vi "DrawSeparator.vi"(7 "Collection in":refnum<class "Collection.lvclass">, 8 "error in (no error)":errorcluster, 9 "XPos":i16, 10 "Point":refnum<class "Point.lvclass">, 11 "Menu in":refnum<class "Menu.lvclass">) -> (0 "error out":errorcluster, 2 "rect":T1, 3 "Menu out":refnum<class "Menu.lvclass">, 5 "Collection out":refnum<class "Collection.lvclass">)   [LabVIEW 2021, in "Menu.lvlib" / "Menu.lvclass"]
uses:
  Menu.lvclass
  Picture2D/src/Point/Point.lvclass
  Picture2D/src/Collection/Collection.lvclass
  Picture2D/src/Line/Line.lvclass
  C:/GitHub/Picture2D/src/Shape/Shape.lvclass
  C:/GitHub/Picture2D/src/IDrawable/IDrawable.lvclass
  Picture2D/src/Text/Text.lvclass
  C:/GitHub/Picture2D/src/Picture2D/Picture2D.lvclass
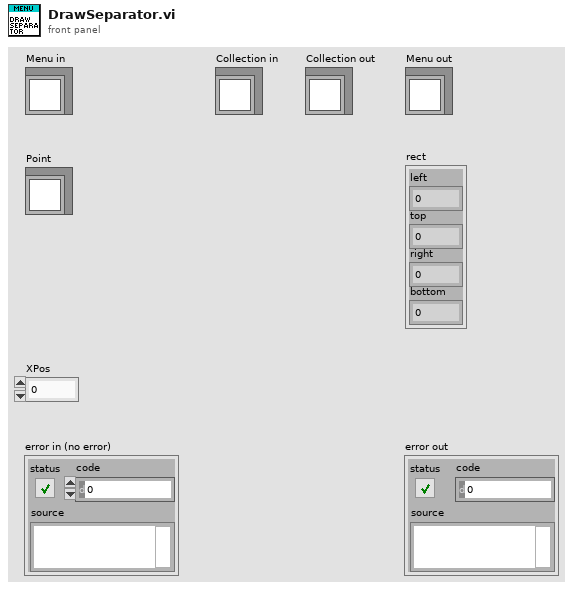
[diagram p1: front panel]
types:
  T1 = cluster{"left":i16, "top":i16, "right":i16, "bottom":i16}
  T2 = typedef "Menu.lvlib/Menu.lvclass/MenuColors.ctl" = cluster{"Text":refnum<class "Color.lvclass">, "HiliteText":refnum<class "Color.lvclass">, "Background":refnum<class "Color.lvclass">, "BorderColor":refnum<class "Color.lvclass">, "Hilite":refnum<class "Color.lvclass">}
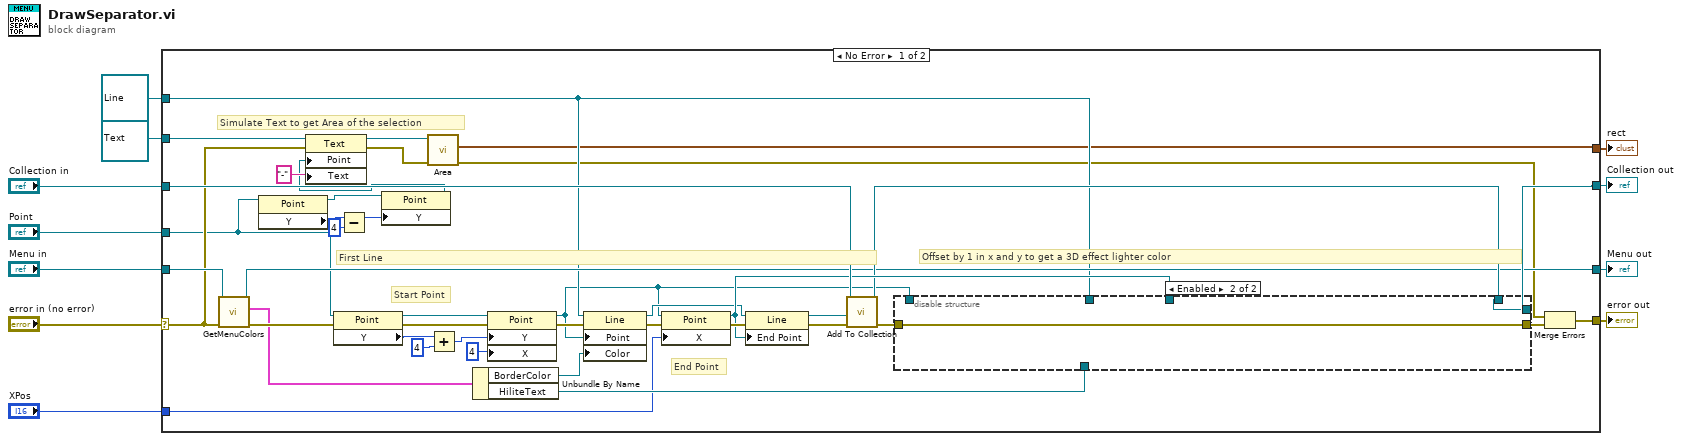
[diagram p0: block diagram]
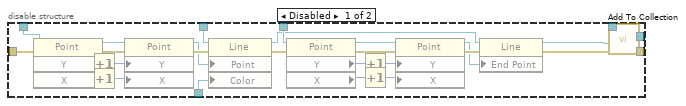
[diagram p2: hidden frame]
diagram:
  n1 = case shown="No Error" "error in (no error)" {
    selector: "error in (no error)" -> [w27 w83]
    tunnel: [w25 w83] -> w11
    tunnel: "XPos" -> [w45 _]
    tunnel: "Point" -> [w17 _]
    tunnel: [w19 _] -> w8
    tunnel: "Collection in" -> [w39 w84]
    tunnel: [w38 w84] -> w6
    tunnel: [w32 w85] -> w4
    tunnel: "Menu in" -> [w31 w85]
    tunnel: refnum<class "Line.lvclass"> refnum ("Picture2D.lvlib:Line") -> [w29 _]
    tunnel: refnum<class "Text.lvclass"> refnum ("Picture2D.lvlib:Text") -> [w28 _]
    frame No Error {
      # "End Point"
      # "Start Point"
      # "Simulate Text to get Area of the selection"
      # "First Line"
      # "Offset by 1 in x and y to get a 3D effect lighter color"
      n2 = call "GetMenuColors.vi"("error in (no error)"=w27, "Menu in"=w31) -> ("error out"=w33:errorcluster, "MenuColors"=w30:T2, "Menu out"=w32:refnum<class "Menu.lvclass">)  [unwired: 7 in]
      n3 = property class="Point"(reference=w17) -> (reference out=w15:refnum<class "Point.lvclass">, "Y"=w16:i16)  [unwired: 1 in, 1 out]
      n4 = property class="Point"(reference=w17, error in=w33) -> (reference out=w41:refnum<class "Point.lvclass">, error out=w48:errorcluster, "Y"=w42:i16)
      n5 = Subtract(x=w16, y=i16 4) -> (x-y=w13:i16)
      n6 = property class="Point"(reference=w15, "Y"=w13) -> (reference out=w14:refnum<class "Point.lvclass">)  [unwired: 1 in, 1 out]
      n7 = property class="Text"(reference=w28, error in=w27, "Point"=w14, "Text"="-") -> (reference out=w40:refnum<class "Text.lvclass">, error out=w26:errorcluster)
      n8 = call-dynamic "Area.vi"("error in (no error)"=w26, "Text in"=w40) -> ("error out"=w24:errorcluster, "rect"=w19:T1)  [unwired: 7 in, 1 out]
      n9 = Add(x=w42, y=i16 4) -> (x+y=w43:i16)
      n10 = Unbundle By Name(w30) -> ("BorderColor"=w21:refnum<class "Color.lvclass">, "HiliteText"=w47:refnum<class "Color.lvclass">)
      n11 = property class="Point"(reference=w41, error in=w48, "Y"=w43, "X"=i16 4 ("Point:x")) -> (reference out=w18:refnum<class "Point.lvclass">, error out=w49:errorcluster)
      n12 = property class="Line"(reference=w29, error in=w49, "Point"=w18, "Color"=w21) -> (reference out=w35:refnum<class "Line.lvclass">, error out=w50:errorcluster)
      n13 = property class="Point"(reference=w18, error in=w50, "X"=w45) -> (reference out=w37:refnum<class "Point.lvclass">, error out=w51:errorcluster)
      n14 = property class="Line"(reference=w35, error in=w51, "End Point"=w37) -> (reference out=w20:refnum<class "Line.lvclass">, error out=w23:errorcluster)
      n15 = call-dynamic "Add To Collection.vi"("error in (no error)"=w23, "IDrawable"=w20, "Collection in"=w39) -> ("error out"=w22:errorcluster, "Collection out"=w36:refnum<class "Collection.lvclass">)  [unwired: 7 in]
      n16 = disable-structure shown="Enabled" {
        disable-tunnel: [w80 w81] -> w52
        disable-tunnel: w47 -> [w74 _]
        disable-tunnel: w18 -> [w73 _]
        disable-tunnel: [w72 w82] -> w38
        disable-tunnel: w37 -> [w71 _]
        disable-tunnel: w36 -> [w56 w82]
        disable-tunnel: w29 -> [w55 _]
        disable-tunnel: w22 -> [w54 w81]
        frame Disabled {
          n17 = property class="Point"(reference=w73, error in=w54) -> (reference out=w60:refnum<class "Point.lvclass">, error out=w75:errorcluster, "Y"=w59:i16, "X"=w61:i16)
          n18 = Increment(x=w59) -> (x+1=w63:i16)
          n19 = Increment(x=w61) -> (x+1=w62:i16)
          n20 = property class="Point"(reference=w60, error in=w75, "Y"=w63, "X"=w62) -> (reference out=w64:refnum<class "Point.lvclass">, error out=w76:errorcluster)
          n21 = property class="Line"(reference=w55, error in=w76, "Point"=w64, "Color"=w74) -> (reference out=w57:refnum<class "Line.lvclass">, error out=w77:errorcluster)
          n22 = property class="Point"(reference=w71, error in=w77) -> (reference out=w68:refnum<class "Point.lvclass">, error out=w78:errorcluster, "Y"=w69:i16, "X"=w67:i16)
          n23 = Increment(x=w69) -> (x+1=w65:i16)
          n24 = Increment(x=w67) -> (x+1=w66:i16)
          n25 = property class="Point"(reference=w68, error in=w78, "Y"=w65, "X"=w66) -> (reference out=w70:refnum<class "Point.lvclass">, error out=w79:errorcluster)
          n26 = property class="Line"(reference=w57, error in=w79, "End Point"=w70) -> (reference out=w58:refnum<class "Line.lvclass">, error out=w53:errorcluster)
          n27 = call-dynamic "Add To Collection.vi"("error in (no error)"=w53, "IDrawable"=w58, "Collection in"=w56) -> ("error out"=w80:errorcluster, "Collection out"=w72:refnum<class "Collection.lvclass">)  [unwired: 7 in]
        }
        frame Enabled {
        }
      }
      n28 = Merge Errors(w24, w52) -> (w25:errorcluster)
    }
    frame Error {
    }
  }
  "Menu out" <- w4
  "error out" <- w11
  "rect" <- w8
  "Collection out" <- w6
